vi "DegtoPWM.vi"(10 "Desired Angle":dbl(slide) scale=-90.0..90.0, 11 "PWM Frequency":dbl=50.0) -> (3 "PWM Output":dbl)   [LabVIEW 2014]
panel:
  out "msec Output":dbl
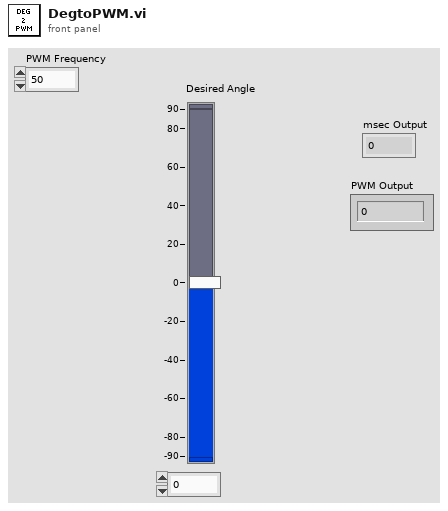
[diagram p1: front panel]
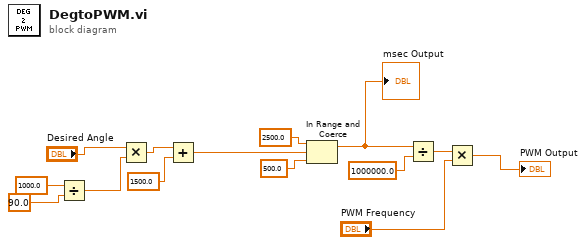
[diagram p0: block diagram]
diagram:
  n1 = Divide(x=1000.0, y=90.0) -> (x/y=w5:dbl)
  n2 = Multiply(x="Desired Angle", y=w5) -> (x*y=w4:dbl)
  n3 = Add(x=w4, y=1500.0) -> (x+y=w2:dbl)
  n4 = In Range and Coerce(upper limit=2500.0, x=w2, lower limit=500.0) -> (coerced(x)=w12:dbl)  [unwired: 1 out]
  "msec Output" <- w12
  n5 = Divide(x=w12, y=1000000.0) -> (x/y=w13:dbl)
  n6 = Multiply(x=w13, y="PWM Frequency") -> (x*y=→"PWM Output":dbl)
